vi "PicoScope3000aExampleBlock_AdvancedTrig.vi"() -> ()   [LabVIEW 2016]
uses:
  <vilib>/Waveform/DWDTOps.llb/DWDT Analog to Digital.vi
  PicoScope3000aLib/PicoScope3000aAnalogChannelSettings.ctl
  PicoScope3000aLib/PicoScope3000aDigitalChannelSettings.ctl
panel:
  out "Channel A":T1(graph)
  out "overflow":i16 format="%08b"
  in  "Acquisition Settings":T2={"preTriggerSamples"=0, "postTriggerSamples"=1000, "timebase"=2, "Down-Sample Mode"=0, "Down Sample Ratio"=1} {"Down Sample Ratio" min=1 step=1; "Down-Sample Mode" items=["None"=0, "Aggregate"=1, "Decimate"=2, "Average"=4]}
  in  "Channel A Settings":T3={"Enabled"=TRUE, "Coupling"=1, "Range"=6, "Analogue Offset"=0.0, "Bandwidth Limit"=0} {"Bandwidth Limit" items=["Full", "20MHz"]; "Range" items=["10 mV", "20 mV", "50 mV", "100 mV", "200 mV", "500 mV", "1 V", "2 V", "5 V", "10 V", "20 V", "50 V ", "100 V"]; "Coupling" items=["AC", "DC"]}
  in  "Port 0 Settings":T4={"Enabled"=FALSE, "Logic Level"=9830} {"Logic Level" items=["1.5V TTL"=9830, "2.5V CMOS"=16383]}
  in  "Digital Port  0":T5 {"Direction Channel 7" items=["Don't Care", "Low", "High", "Rising", "Falling"]; "Direction Channel 6" items=["Don't Care", "Low", "High", "Rising", "Falling"]; "Direction Channel 5" items=["Don't Care", "Low", "High", "Rising", "Falling"]; "Direction Channel 4" items=["Don't Care", "Low", "High", "Rising", "Falling"]; "Direction Channel 3" items=["Don't Care", "Low", "High", "Rising", "Falling"]; "Direction Channel 2" items=["Don't Care", "Low", "High", "Rising", "Falling"]; "Direction Channel 1" items=["Don't Care", "Low", "High", "Rising", "Falling"]; "Direction Channel 0" items=["Don't Care", "Low", "High", "Rising", "Falling"]}
  in  "Trigger Conditions":T6={"Channel A"=TRUE, "Channel B"=FALSE, "Channel C"=FALSE, "Channel D"=FALSE, "Aux"=FALSE, "PWQ"=FALSE, "Condition Logic"=0, "Ext"=FALSE, "Digital"=FALSE} {"Condition Logic" items=["AND", "OR", "XOR"]}
  in  "Channel A Trigger Properties":T7={"thresholdUpper"=0, "thresholdUpperHysteresis"=0, "thresholdLower"=0, "thresholdLowerHysteresis"=0, "Threshold Mode"=0, "Direction"=0, "Available"=TRUE} {"Direction" items=["Above / Inside", "Below / Outside", "Rising / Enter", "Falling / Exit", "Rising or Falling / Enter or Exit", "Above Lower", "Below Lower", "Rising Lower", "Falling Lower", "Positive Runt", "Negative Runt"]; "Threshold Mode" items=["Level", "Window"]}
  out "Port 0 Digital Waveform Graph":digitalwaveform(graph)
  in  "stop":bool
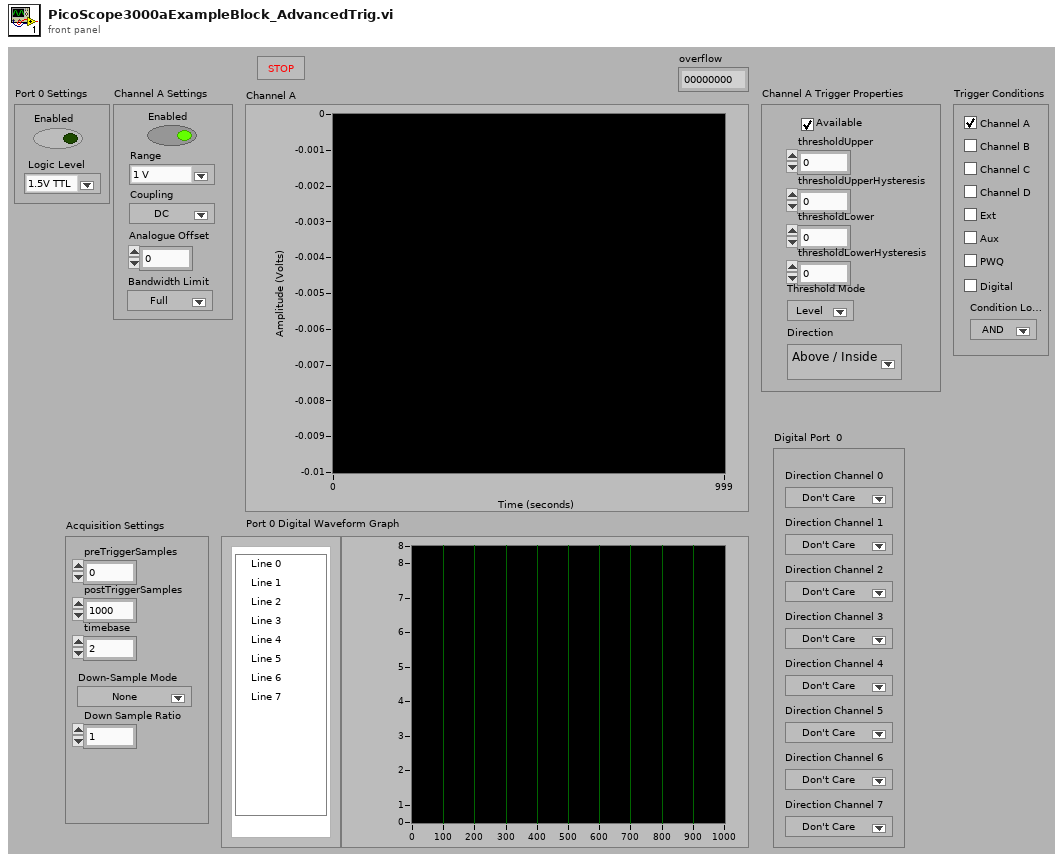
[diagram p1: front panel]
types:
  T1 = cluster{i32, "full-scale range (pk-pk)":dbl, "Data":dbl[]}
  T2 = cluster{"preTriggerSamples":u32, "postTriggerSamples":u32, "timebase":u32, "Down-Sample Mode":i32, "Down Sample Ratio":u32}
  T3 = typedef "PicoScope3000aAnalogChannelSettings.ctl" = cluster{"Enabled":bool, "Coupling":u32, "Range":u32, "Analogue Offset":sgl, "Bandwidth Limit":u32}
  T4 = typedef "PicoScope3000aDigitalChannelSettings.ctl" = cluster{"Enabled":bool, "Logic Level":i16}
  T5 = cluster{"Direction Channel 0":u16, "Direction Channel 1":u16, "Direction Channel 2":u16, "Direction Channel 3":u16, "Direction Channel 4":u16, "Direction Channel 5":u16, "Direction Channel 6":u16, "Direction Channel 7":u16}
  T6 = cluster{"Channel A":bool, "Channel B":bool, "Channel C":bool, "Channel D":bool, "Aux":bool, "PWQ":bool, "Condition Logic":u16, "Ext":bool, "Digital":bool}
  T7 = cluster{"thresholdUpper":i16, "thresholdUpperHysteresis":u16, "thresholdLower":i16, "thresholdLowerHysteresis":u16, "Threshold Mode":i32, "Direction":i32, "Available":bool}
  T8 = cluster{"Driver Version":string, "USB Version":string, "Hardware":string, "Variant":string, "Batch and Serial":string, "Cal Date":string, "Kernel Version":string, "Digital HW Version":string, "Analogue HW Version":string, "MSO":bool, "Number of channels":i16}
  T9 = cluster{"Channel D Buffer":i16[], "Channel C Buffer":i16[], "Channel B Buffer":i16[], "Channel A Buffer":i16[], "Port 0  Buffer ":i16[], "Port 1 Buffer ":i16[]}
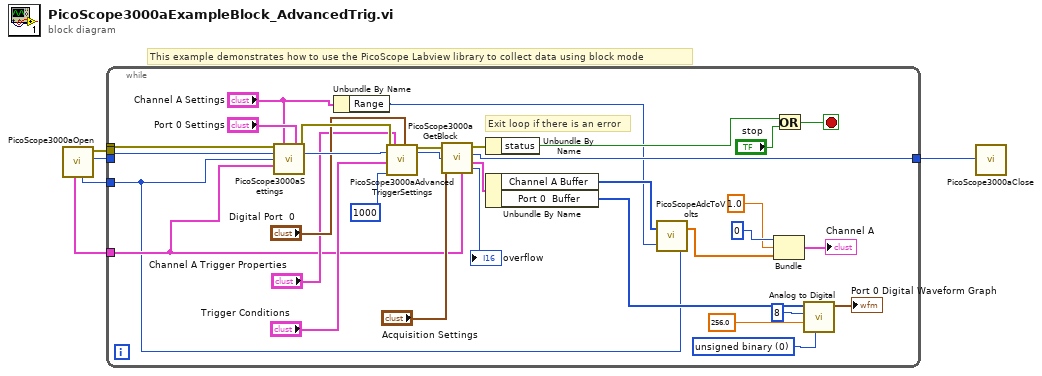
[diagram p0: block diagram]
diagram:
  # "This example demonstrates how to use the PicoScope Labview library to collect data using block mode"
  n1 = call "PicoScope3000aOpen.vi"() -> ("handle"=w4:i16, "error out"=w5:errorcluster, "Max ADC value"=w1:i16, "Device Info"=w2:T8)  [unwired: 6 in, 2 out]
  n2 = while {
    tunnel: w4 -> [w30]
    tunnel: [w18] -> _
    tunnel: [w28] -> w3
    tunnel: w5 -> [w18]
    tunnel: w2 -> [w15]
    tunnel: w1 -> [w9]
    stop <- w38 stop-if-true
    w34 = u16 0 items=["unsigned binary", "offset binary", "2's complement"] ("data format (offset binary)")
    # "Exit loop if there is an error"
    n3 = call "PicoScope3000aSettings.vi"("error in"=w18, "Channel A Settings"="Channel A Settings", "Port 0 Settings"="Port 0 Settings", "handle in"=w30, "Max_adc"=w9, "Device Info"=w15) -> ("error out"=w26:errorcluster, "handle out"=w25:i16)  [unwired: 7 in, 1 out]
    n4 = Unbundle By Name("Channel A Settings") -> ("Range"=w8:u32)
    n5 = call "PicoScope3000aAdvancedTriggerSettings.vi"("error in"=w26, "handle in"=w25, "Trigger Conditions"="Trigger Conditions", "Auto Trigger (ms)"=1000, "Channel A Trigger Properties"="Channel A Trigger Properties", "Digital Port  0"="Digital Port  0") -> ("error out"=w21:errorcluster, "handle out"=w20:i16)  [unwired: 12 in]
    n6 = call "PicoScope3000aGetBlock.vi"("error in"=w21, "handle in"=w20, "Acquisition Settings"="Acquisition Settings", "Device Info"=w15) -> ("overflow"=→"overflow":i16, "error out"=w27:errorcluster, "handle out"=w28:i16, "Buffers (Max or non-aggregated)"=w29:T9)  [unwired: 1 in, 2 out]
    n7 = Unbundle By Name(w27) -> ("status"=w36:bool)
    n8 = Unbundle By Name(w29) -> ("Channel A Buffer"=w10:i16[], "Port 0  Buffer"=w31:i16[])
    n9 = call "PicoScopeAdcToVolts.vi"("Max_adc"=w9, "Range Index"=w8, "Data"=w10) -> ("Data"=w11:dbl[])
    n10 = Bundle(0, "full-scale range (pk-pk)"=1.0, "Data"=w11) -> (→"Channel A":T1)  [unwired: 1 in]
    n11 = Or(x=w36, y="stop") -> (x .or. y?=w38:bool)
    n12 = call-poly <vilib>:"Analog to Digital.vi"("data format (offset binary)"=w34, "full-scale range (pk-pk)"=256.0, "resolution (16 bit)"=8, "analog waveform"=w31) -> ("digital waveform"=→"Port 0 Digital Waveform Graph":digitalwaveform)  [unwired: 4 in, 3 out]
  }
  n13 = call "PicoScope3000aClose.vi"("handle"=w3) -> ()
